vi "worksheet split panes opt.vi"(6 "left_col":u16, 7 "top_row":u32, 8 "error in (no error)":errorcluster, 9 "horizontal":dbl, 10 "vertical":dbl, 11 "worksheet":u32) -> (0 "error out":errorcluster)   [LabVIEW 8.6]
doc: "void worksheet_split_panes_opt(lxw_worksheet worksheet, double vertical, double horizontal, lxw_row_t top_row, lxw_col_t left_col);"
uses:
  pending_lvxlsxwriter/xlsxwriter.dll
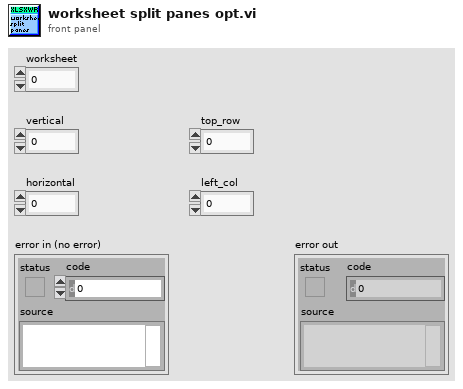
[diagram p1: front panel]
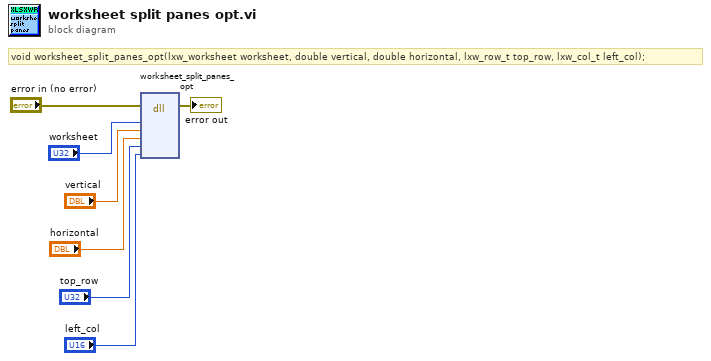
[diagram p0: block diagram]
diagram:
  # "void worksheet_split_panes_opt(lxw_worksheet worksheet, double vertical, double horizontal, lxw_row_t top_row, lxw_col_t left_col);"
  n1 = dll-call lib="C:/Users/WDAGUtilityAccount/Desktop/pending_lvxlsxwriter/xlsxwriter.*" fn="worksheet_split_panes_opt"(error in="error in (no error)", "worksheet"="worksheet", "vertical"="vertical", "horizontal"="horizontal", "top_row"="top_row", "left_col"="left_col") -> (error out=→"error out":errorcluster)  [unwired: 8 in, 1 out]
